vi "MOTmasterfilesort.vi"() -> ()   [LabVIEW 2016]
uses:
  <vilib>/regexp/Match Regular Expression.xnode
panel:
  out "size(s) 2":i32
  out "Array 2":string[](array[string])
  out "match + rest of string":string
  out "size(s)":i32
  out "Array":i32[](array[numeric])
  in  "file (use dialog)":path
  out "text":string
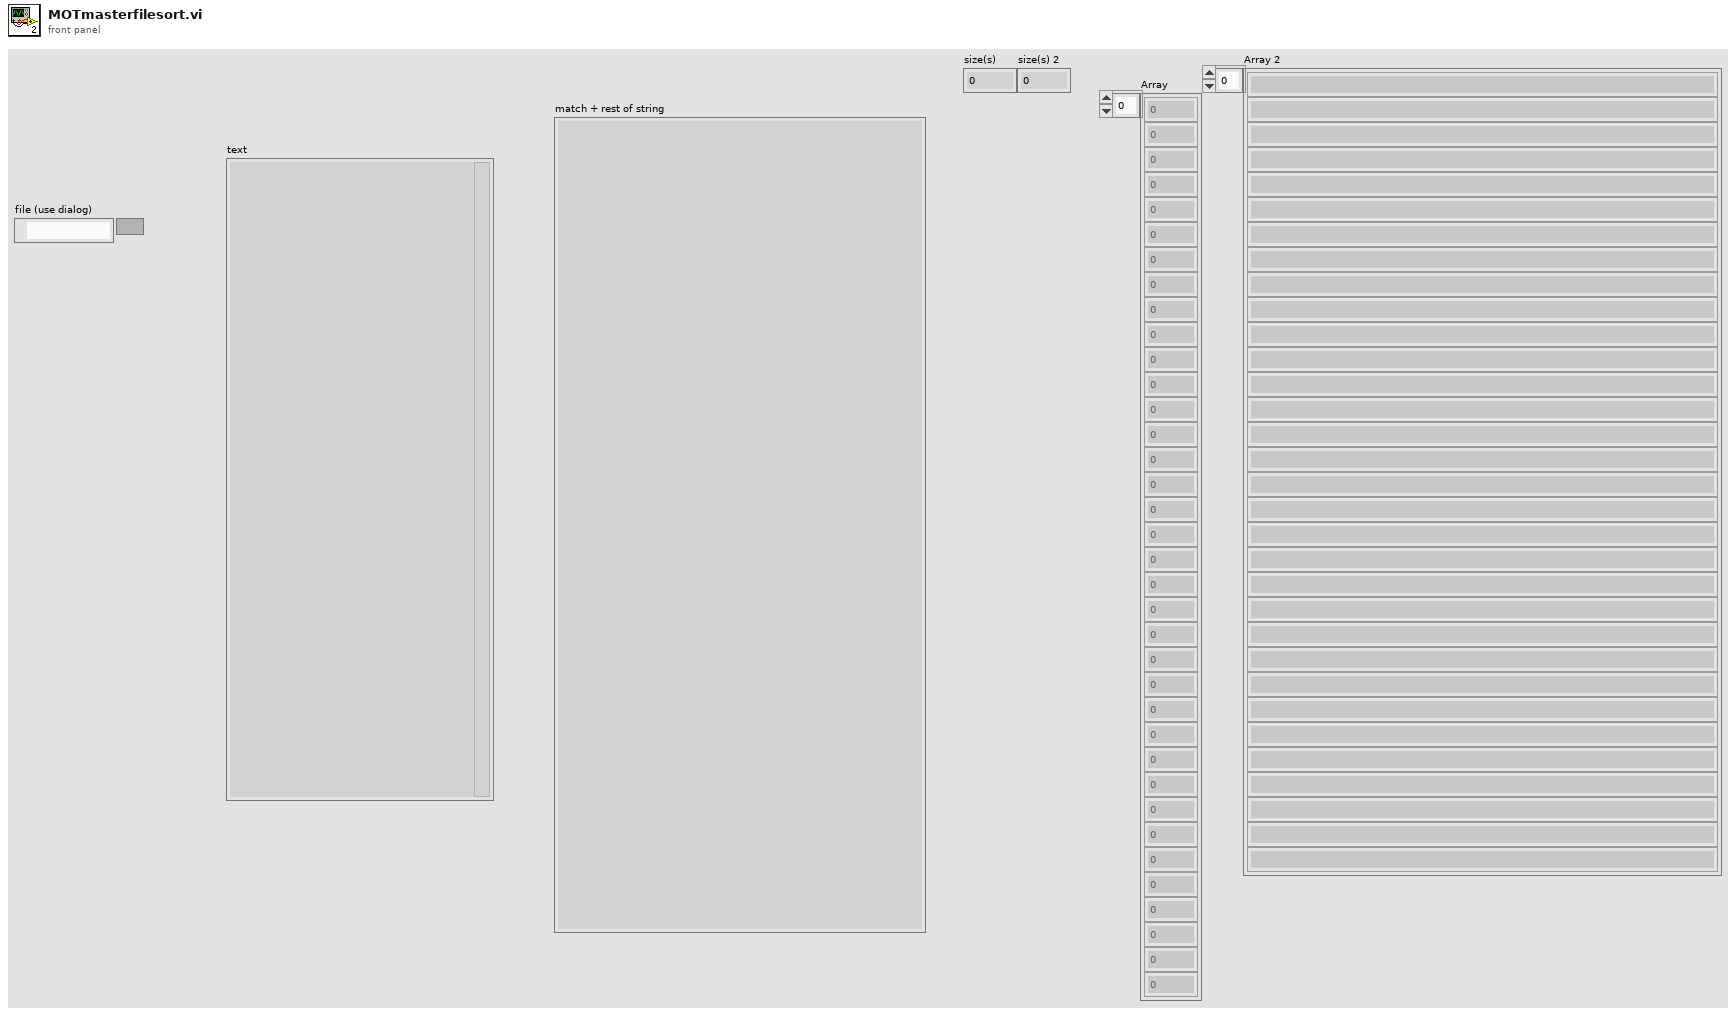
[diagram p1: front panel]
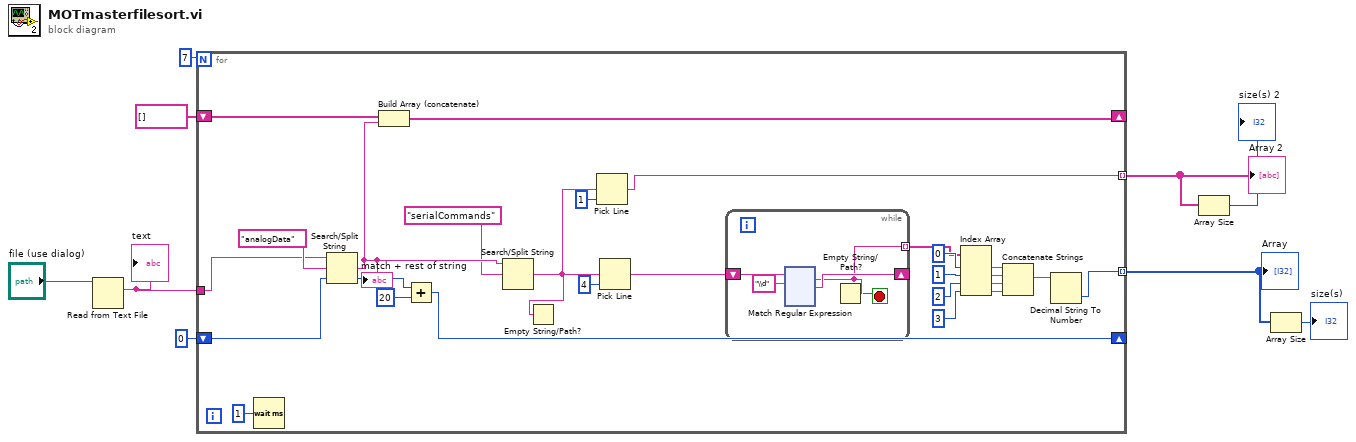
[diagram p0: block diagram]
diagram:
  n1 = Read from Text File(file (use dialog)="file (use dialog)") -> (text=w7:string)  [unwired: 3 in, 3 out]
  "text" <- w7
  n2 = for {
    N: 7 -> [_]
    shift-right: [w29] -> _
    shift-left: string[] [] -> [w28]
    shift-right: [w33] -> _
    shift-left: 0 -> [w32]
    tunnel: w7 -> [w30]
    tunnel: [w13] -> w5 mode=indexing
    tunnel: [w10] -> w3 mode=indexing
    n3 = Wait (ms)(milliseconds to wait=u32 1) -> ()  [unwired: 1 out]
    n4 = Search/Split String(string=w30, search string/char (-)="analogData", offset (0)=w32) -> (match + rest of string=w27:string, offset of match=w35:i32)  [unwired: 1 out]
    "match + rest of string" <- w27
    n5 = Build Array (concatenate)(w28, w27) -> (w29:string[])
    n6 = Add(x=w35, y=20) -> (x+y=w33:i32)
    n7 = Search/Split String(string=w27, search string/char (-)="serialCommands") -> (match + rest of string=w12:string)  [unwired: 1 in, 2 out]
    n8 = Empty String/Path?(string/path=w12) -> ()  [unwired: 1 out]
    n9 = Pick Line(multi-line string=w12, line index=1) -> (output string=w10:string)  [unwired: 1 in]
    n10 = Pick Line(multi-line string=w12, line index=4) -> (output string=w15:string)  [unwired: 1 in]
    n11 = while {
      shift-right: [w40] -> _
      shift-left: w15 -> [w41]
      tunnel: [w39] -> w16 mode=indexing
      stop <- w38 stop-if-true
      n12 = xnode "Match Regular Expression"("input string"=w41, "regular expression"="\\d") -> ("whole match"=w39:string, "after match"=w40:string)  [unwired: 4 in, 3 out]
      n13 = Empty String/Path?(string/path=w39) -> (empty?=w38:bool)
    }
    n14 = Index Array(array=w16, index #1=0 ("index"), index #2=1 ("index"), index #3=2 ("index"), index #4=3 ("index")) -> (element #1=w21:string, element #2=w22:string, element #3=w23:string, element #4=w24:string)
    n15 = Concatenate Strings(w21, w22, w23, w24) -> (w14:string)
    n16 = Decimal String To Number(string=w14) -> (number=w13:i32)  [unwired: 2 in, 1 out]
  }
  "Array" <- w5
  "Array 2" <- w3
  n17 = Array Size(array=w3) -> (size(s)=→"size(s) 2":i32)
  n18 = Array Size(array=w5) -> (size(s)=→"size(s)":i32)
